vi "Digital Read Multiple Channels.vi"(8 "error in (no error)":errorcluster, 10 "Array":i32[](array[numeric]), 11 "NI-DAQ in":refnum<class "NI-DAQ.lvclass">) -> (0 "error out":errorcluster, 2 "subarray":bool[](array[boolean]), 3 "NI-DAQ out":refnum<class "NI-DAQ.lvclass">)   [LabVIEW 2021, in "NI-DAQ.lvclass"]
uses:
  NI-DAQ.lvclass
  NI-DAQ.lvclass/NI-DAQ.ctl
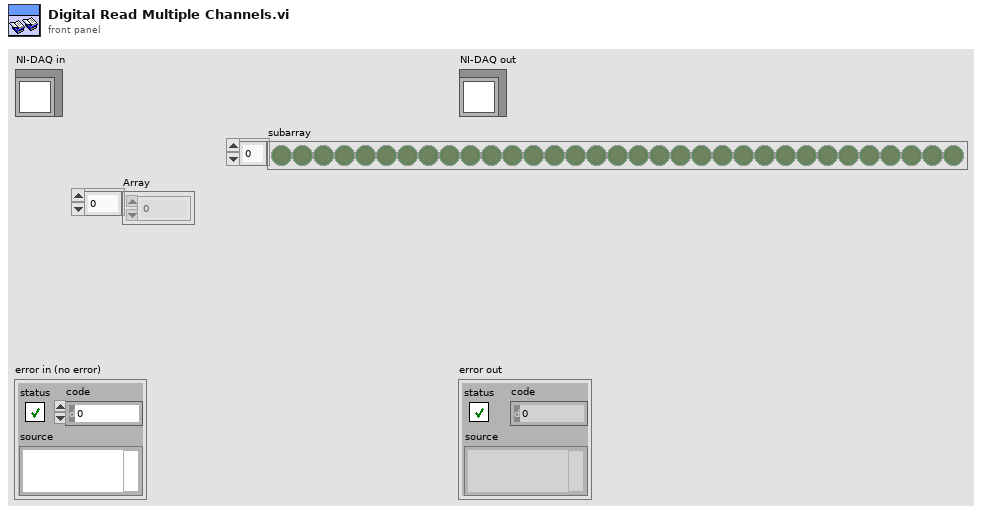
[diagram p1: front panel]
types:
  T1 = typedef "I-O.lvclass/Pin Map.ctl" = cluster{"Region Valves":i32[], "Extra Valves":dbl[][][], "Tool Primary Valve":i32, "Tool Secondary Valve":i32, "Region Sensors":i32[], "Extra Sensors":dbl[][][], "Tool Primary Sensor":dbl, "Tool Secondary Sensor":dbl, "Compression Sensor":dbl, "5V":i32, "Dispenser Sensor":dbl}
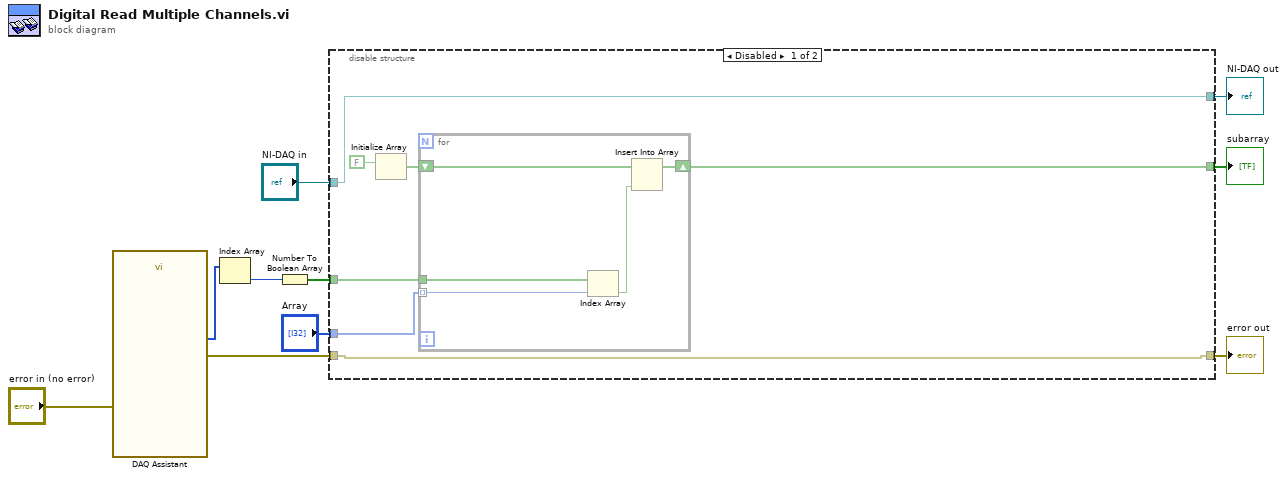
[diagram p0: block diagram]
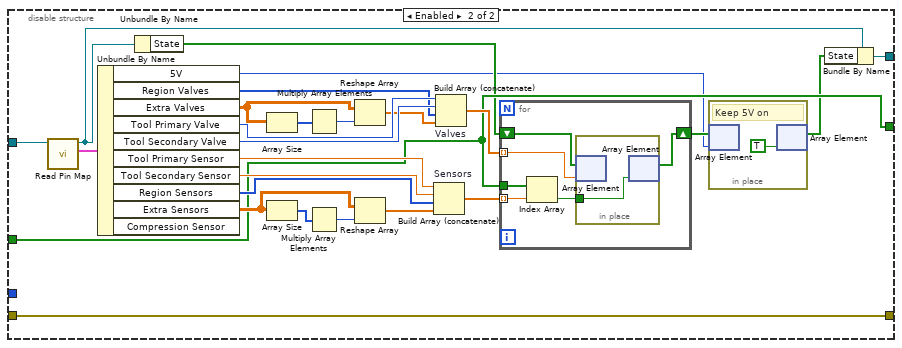
[diagram p2: hidden frame]
diagram:
  n1 = call "DAQ Assistant"("error in"="error in (no error)") -> ("data"=w1:u32[], "error out"=w2:errorcluster)  [unwired: 16 in, 1 out]
  n2 = Index Array(array=w1) -> (element=w10:u32)  [unwired: 1 in]
  n3 = Number To Boolean Array(number=w10) -> (Boolean array=w9:bool[])
  n4 = disable-structure shown="Disabled" {
    disable-tunnel: w9 -> [w17 w27]
    disable-tunnel: "Array" -> [w16 _]
    disable-tunnel: [w13 w27] -> w7
    disable-tunnel: [w12 w48] -> w5
    disable-tunnel: "NI-DAQ in" -> [w12 w46]
    disable-tunnel: [w11 w47] -> w3
    disable-tunnel: w2 -> [w11 w47]
    frame Disabled {
      n5 = Initialize Array(FALSE) -> (w15:bool[])  [unwired: 1 in]
      n6 = for {
        tunnel: w17 -> [w22]
        tunnel: w16 -> [w21] mode=indexing
        shift-right: [w20] -> w13
        shift-left: w15 -> [w19]
        n7 = Index Array(array=w22, index=w21) -> (element=w18:bool)
        n8 = Insert Into Array(array=w19, new element=w18) -> (w20:bool[])  [unwired: 1 in]
      }
    }
    frame Enabled {
      n9 = call-dynamic "Read Pin Map.vi"("NI-DAQ in"=w46) -> ("Pin Map"=w45:T1, "NI-DAQ out"=w44:refnum<class "NI-DAQ.lvclass">)  [unwired: 8 in, 1 out]
      n10 = Unbundle By Name(w45) -> ("5V"=w24:i32, "Region Valves"=w41:i32[], "Extra Valves"=w38:dbl[][][], "Tool Primary Valve"=w43:i32, "Tool Secondary Valve"=w42:i32, "Tool Primary Sensor"=w34:dbl, "Tool Secondary Sensor"=w33:dbl, "Region Sensors"=w32:i32[], "Extra Sensors"=w31:dbl[][][])  [unwired: 1 out]
      n11 = Unbundle By Name(w44) -> ("State"=w26:bool[])
      n12 = Array Size(array=w38) -> (size(s)=w40:i32[])
      n13 = Array Size(array=w31) -> (size(s)=w36:i32[])
      n14 = Multiply Array Elements(1:w40) -> (0:w39:i32)
      n15 = Multiply Array Elements(1:w36) -> (0:w35:i32)
      n16 = Reshape Array(w38, w39) -> (w37:dbl[])
      n17 = Reshape Array(w31, w35) -> (w30:dbl[])
      n18 = Build Array (concatenate) "Sensors"(w34, w33, w32, w30) -> (w28:dbl[])
      n19 = Build Array (concatenate) "Valves"(w43, w42, w41, w37) -> (w29:dbl[])
      n20 = for {
        tunnel: w28 -> [w50] mode=indexing
        tunnel: w27 -> [w54]
        shift-right: [w52] -> w25
        shift-left: w26 -> [w53]
        tunnel: w29 -> [w49] mode=indexing
        n21 = Index Array(array=w54, index=w50) -> (element=w51:bool)
        n22 = in-place {
          in-place-border: w51 -> [w55]
          n23 = in-place-array #1(w53, w49) -> ()  [unwired: 1 out]
          n24 = in-place-array #1(w55) -> (w52:bool[])  [unwired: 1 out]
        }
      }
      n25 = in-place {
        # "Keep 5V on"
        n26 = in-place-array #2(w25, w24) -> ()  [unwired: 1 out]
        n27 = in-place-array #2(TRUE ("element")) -> (w23:bool[])  [unwired: 1 out]
      }
      n28 = Bundle By Name(cluster=w44, "State"=w23) -> (w48:refnum<class "NI-DAQ.lvclass">)
    }
  }
  "error out" <- w3
  "NI-DAQ out" <- w5
  "subarray" <- w7
